vi "SigProcOptions.vi"(0 "Compress":bool, 1 "Chirp Filter":cluster{"Spectrum":cdb[], "Size":i32}, 2 "sample rate MHz":i32, 3 "Data In":dbl[][](array[numeric]), 5 "Filter Prams":T1={"Filter"=FALSE, "low cutoff"=5, "order"=81, "high cutoff"=35}) -> (6 "Data Out":dbl[][](array[numeric]))   [LabVIEW 2022 SP3]
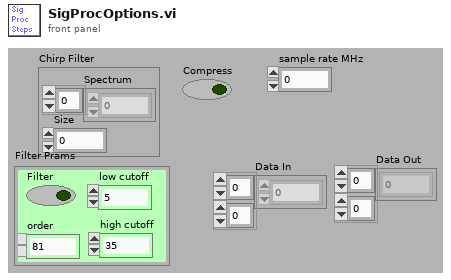
[diagram p1: front panel]
types:
  T1 = cluster{"Filter":bool, "low cutoff":i32, "order":i32, "high cutoff":i32}
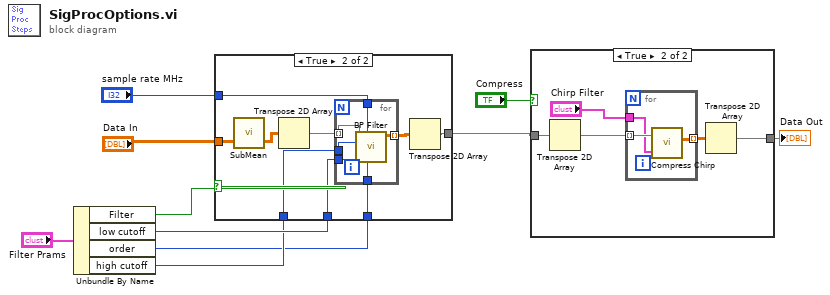
[diagram p0: block diagram]
diagram:
  n1 = Unbundle By Name("Filter Prams") -> ("Filter"=w5:bool, "low cutoff"=w4:i32, "order"=w2:i32, "high cutoff"=w3:i32)
  n2 = case shown="True" w5 {
    tunnel: [w11 w19] -> w8
    tunnel: "Data In" -> [w11 w16]
    tunnel: "sample rate MHz" -> [_ w17]
    tunnel: w4 -> [_ w14]
    tunnel: w3 -> [_ w13]
    tunnel: w2 -> [_ w12]
    frame False {
    }
    frame True {
      n3 = call "SubMean.vi"("Scan Data In"=w16) -> ("Array"=w15:dbl[][])  [unwired: 1 in, 1 out]
      n4 = Transpose 2D Array(2D array=w15) -> (transposed array=w18:dbl[][])
      n5 = for {
        tunnel: [w26] -> w20 mode=indexing
        tunnel: w12 -> [w25]
        tunnel: w14 -> [w24]
        tunnel: w13 -> [w23]
        tunnel: w18 -> [w22] mode=indexing
        tunnel: w17 -> [w21]
        n6 = call "BP Filter.vi"(1:w25, "sample rate MHz"=w21, 3:w24, "Filter Prams"=w23, "Array in"=w22) -> ("Filtered X"=w26:dbl[][])  [unwired: 1 in]
      }
      n7 = Transpose 2D Array(2D array=w20) -> (transposed array=w19:dbl[][])
    }
  }
  n8 = case shown="True" "Compress" {
    tunnel: [w27 w30] -> w7
    tunnel: w8 -> [w27 w29]
    frame False {
    }
    frame True {
      n9 = Transpose 2D Array(2D array=w29) -> (transposed array=w32:dbl[][])
      n10 = for {
        tunnel: w32 -> [w35] mode=indexing
        tunnel: [w34] -> w31 mode=indexing
        tunnel: "Chirp Filter" -> [w33]
        n11 = call "Compress Chirp.vi"("Chirp"=w33, "Array In"=w35) -> ("Array Out"=w34:dbl[][])
      }
      n12 = Transpose 2D Array(2D array=w31) -> (transposed array=w30:dbl[][])
    }
  }
  "Data Out" <- w7
